vi "Pull Stream.vi"(8 "error in (no error)":errorcluster, 10 "timeout in ms (-1)":i32, 11 "stream in":refnum<queue>) -> (0 "error out":errorcluster, 2 "element":T1, 3 "queue out":refnum<queue>)   [LabVIEW 2014, in "Sprocket.lvlib"]
uses:
  lib/Sprocket.lvlib
  Action/Action.ctl
  Action/Action Name.ctl
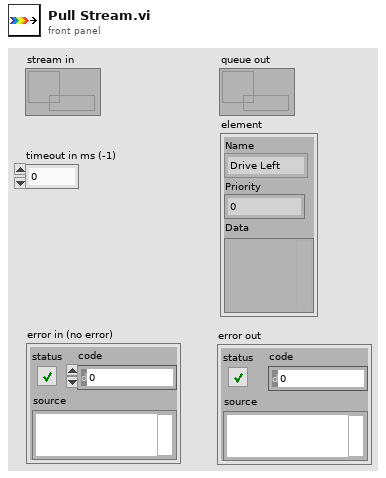
[diagram p1: front panel]
types:
  T1 = typedef "Sprocket.lvlib/Action.ctl" = cluster{"Name":T2, "Priority":i32, "Data":variant}
  T2 = typedef "Sprocket.lvlib/Action Name.ctl" = enum16{"Drive Left", "Drive Right"}
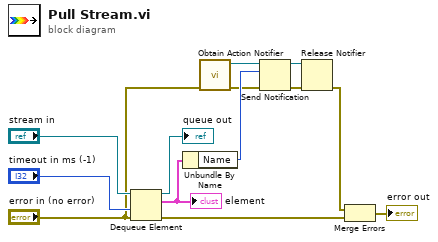
[diagram p0: block diagram]
diagram:
  n1 = Dequeue Element(queue="stream in", timeout in ms (-1)="timeout in ms (-1)", error in (no error)="error in (no error)") -> (queue out=→"queue out":refnum<queue>, element=w8:T1, error out=w2:errorcluster)  [unwired: 1 out]
  "element" <- w8
  n2 = Unbundle By Name(w8) -> ("Name"=w7:T2)
  n3 = call "Obtain Action Notifier.vi"("error in (no error)"="error in (no error)") -> ("error out"=w5:errorcluster, "notifier out"=w10:refnum<notifier>)  [unwired: 9 in]
  n4 = Send Notification(notification=w7, notifier=w10, error in (no error)=w5) -> (notifier out=w9:refnum<notifier>, error out=w6:errorcluster)
  n5 = Release Notifier(notifier=w9, error in (no error)=w6) -> (error out=w3:errorcluster)  [unwired: 1 in, 2 out]
  n6 = Merge Errors(w3, w2) -> (→"error out":errorcluster)
